vi "SUB sum_array.vi"(1 "scale info":variant, 2 "Omega":cluster{"frequency":dbl, "+- f":dbl}, 3 "scalogram matrix":dbl[][](array[numeric])) -> (0 "output waveform":waveform(dbl))   [LabVIEW 2017]
uses:
  <vilib>/addons/_Advanced Signal Processing/NI_AdvSigProcWA.lvlib
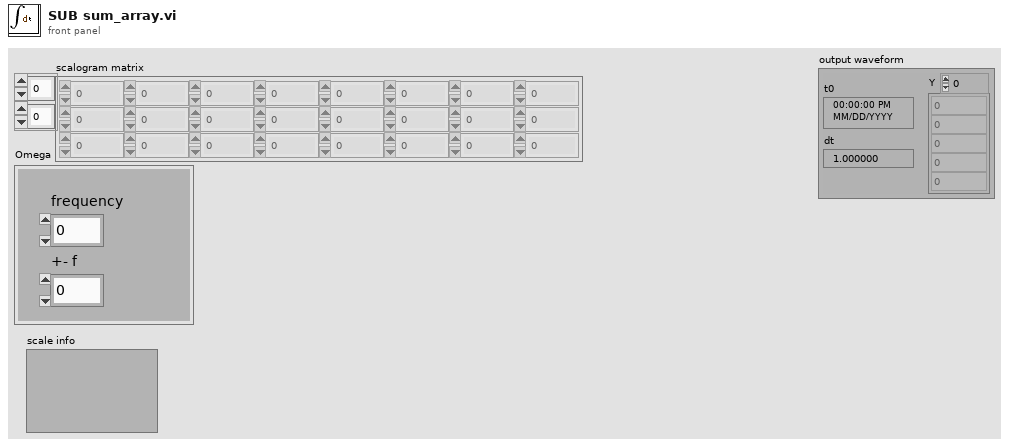
[diagram p1: front panel]
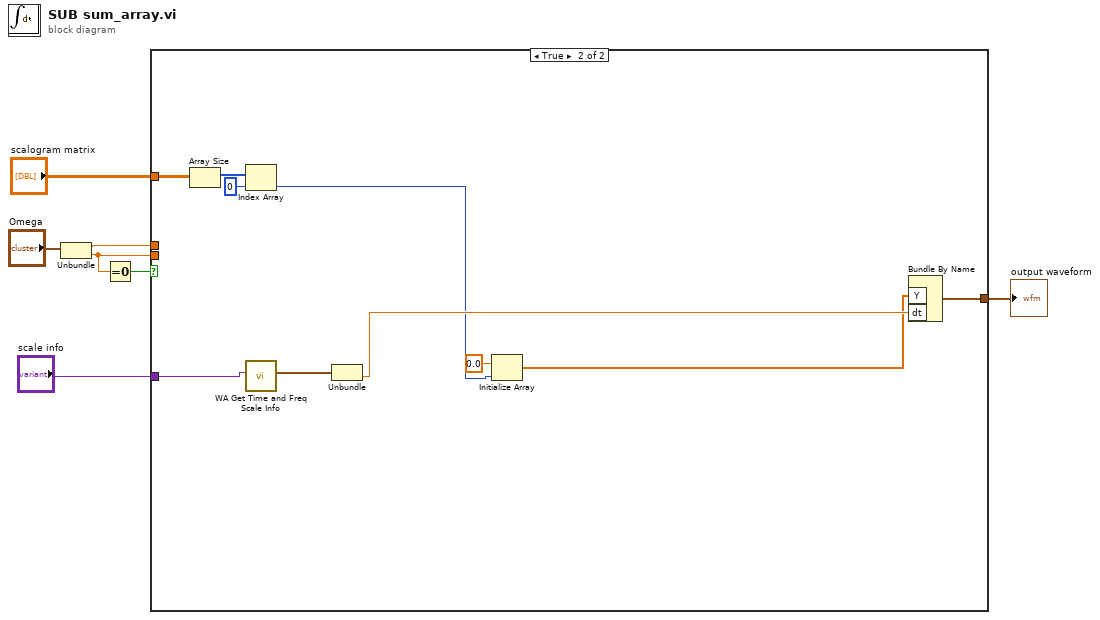
[diagram p0: block diagram]
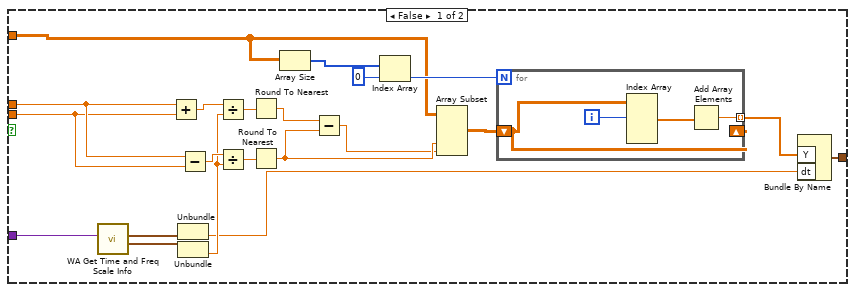
[diagram p2: hidden frame]
diagram:
  n1 = Unbundle("Omega") -> ("frequency"=w4:dbl, "+- f"=w3:dbl)
  n2 = Equal To 0?(x=w3) -> (x = 0?=w5:bool)
  n3 = case shown="True" w5 {
    tunnel: [w13 w39] -> w6
    tunnel: w4 -> [w11 _]
    tunnel: w3 -> [w10 _]
    tunnel: "scalogram matrix" -> [w9 w37]
    tunnel: "scale info" -> [w8 w42]
    frame False {
      n4 = call <vilib>:"WA Get Time and Freq Scale Info.vi"("scale info"=w8) -> ("frequency info"=w28:cluster{"offset":dbl, "multiplier":dbl}, "time info"=w27:cluster{"offset":dbl, "multiplier":dbl})  [unwired: 1 in, 8 out]
      n5 = Add(x=w11, y=w10) -> (x+y=w22:dbl)
      n6 = Unbundle(w27) -> ("multiplier"=w15:dbl)  [unwired: 1 out]
      n7 = Unbundle(w28) -> ("multiplier"=w20:dbl)  [unwired: 1 out]
      n8 = Subtract(x=w11, y=w10) -> (x-y=w26:dbl)
      n9 = Divide(x=w22, y=w20) -> (x/y=w21:dbl)
      n10 = Divide(x=w26, y=w20) -> (x/y=w25:dbl)
      n11 = Round To Nearest(number=w21) -> (nearest integer value=w19:dbl)
      n12 = Round To Nearest(number=w25) -> (nearest integer value=w18:dbl)
      n13 = Array Size(array=w9) -> (size(s)=w24:i32[])
      n14 = Subtract(x=w19, y=w18) -> (x-y=w17:dbl)
      n15 = Index Array(array=w24, index=0) -> (element=w23:i32)
      n16 = Array Subset(array=w9, index (col)=w18, length (col)=w17) -> (w16:dbl[][])  [unwired: 2 in]
      n17 = for {
        N: w23 -> [_]
        shift-right: [w31] -> _
        shift-left: w16 -> [w31]
        tunnel: [w30] -> w14 mode=indexing
        i -> [w29]
        n18 = Index Array(array=w31, index (row) #1=w29) -> (element #1=w32:dbl[])  [unwired: 3 in, 1 out]
        n19 = Add Array Elements(numeric array=w32) -> (sum=w30:dbl)
      }
      n20 = Bundle By Name("Y"=w14, "dt"=w15) -> (w13:waveform(dbl))  [unwired: 1 in]
    }
    frame True {
      n21 = Array Size(array=w37) -> (size(s)=w36:i32[])
      n22 = Index Array(array=w36, index=0) -> (element=w34:i32)
      n23 = call <vilib>:"WA Get Time and Freq Scale Info.vi"("scale info"=w42) -> ("time info"=w41:cluster{"offset":dbl, "multiplier":dbl})  [unwired: 1 in, 9 out]
      n24 = Unbundle(w41) -> ("multiplier"=w38:dbl)  [unwired: 1 out]
      n25 = Initialize Array(0.0 ("element"), w34) -> (w33:dbl[])
      n26 = Bundle By Name("Y"=w33, "dt"=w38) -> (w39:waveform(dbl))  [unwired: 1 in]
    }
  }
  "output waveform" <- w6
